vi "Process.vi"(8 "error in (no error)":errorcluster, 10 "Pound in":refnum<class "Pound.lvclass">, 11 "Qbus in":refnum<class "Qbus.lvclass">) -> (0 "error out":errorcluster)   [LabVIEW 2017, in "CmsAnalysis.lvlib"]
doc: "The Analysis process calculates features and spectral bands, or trends, from waveforms the channels in a data group acquire. After these values are calculated, subsequent processes that evaluate their data to trigger alarms, file collections, and so on can operate."
uses:
  <vilib>/addons/InsightCM/Devices/Shared/Cms/CmsAnalysis/CmsAnalysis.lvlib
  <vilib>/addons/Qbus/Qbus.lvclass
  <vilib>/NI/Software Watchdog/Pound/Pound.lvclass
  <vilib>/addons/InsightCM/Devices/Shared/Cms/CmsAnalysis/controls/Config.ctl
  <vilib>/addons/InsightCM/Devices/Shared/Cms/CmsAnalysis/controls/Group.ctl
  <vilib>/addons/InsightCM/Utilities/Analysis/Shared/controls/Channel.ctl
  <vilib>/addons/InsightCM/Utilities/Analysis/Shared/controls/SpeedType.ctl
  <vilib>/addons/InsightCM/Utilities/Analysis/Shared/controls/Feature.ctl
  <vilib>/addons/InsightCM/Utilities/Analysis/Shared/controls/AmplitudeScale.ctl
  <vilib>/NI/Software Watchdog/Watchdog/Watchdog.lvclass
  <vilib>/addons/InsightCM/Devices/Shared/Common/DataFlow/DataFlow.lvlib
  <vilib>/addons/InsightCM/Utilities/Analysis/Shared/AnalysisHelper.lvlib
  <vilib>/addons/InsightCM/Utilities/GlobalConfiguration/GlobalConfiguration.lvlib
  <vilib>/addons/InsightCM/Devices/Shared/Common/DataEventCreator/DataEventCreator.lvlib
  <vilib>/addons/TraceLogger/TraceLogger.lvlib
  <vilib>/addons/InsightCM/Devices/Shared/Cms/CmsDataEventCreator/CmsDataEventCreator.lvlib
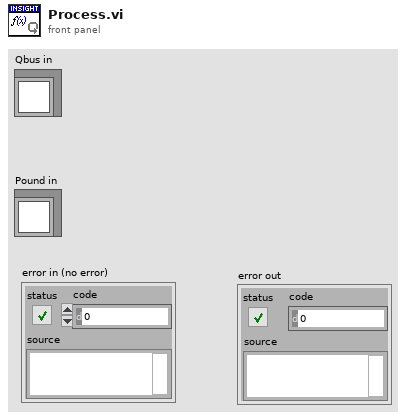
[diagram p1: front panel]
types:
  T1 = typedef "CmsAnalysis.lvlib/Config.ctl" = cluster{"Groups":T2[]}
  T2 = typedef "CmsAnalysis.lvlib/Group.ctl" = cluster{"Name":string, "Channels":T3[]}
  T3 = typedef "AnalysisHelper.lvlib/Channel.ctl" = cluster{"Name":string, "Id":string, "Type":string, "Status Tag":string, "Speed Type":T4, "Speed Reference":string, "Nominal Speed":dbl, "Speed Ratio":dbl, "Pair Channel":string, "Source Channel":string, "Sensitivity":dbl, "Features":T5[], "Acq Timestamp":timestamp}
  T4 = typedef "AnalysisHelper.lvlib/SpeedType.ctl" = enum16{"Fixed Speed", "Tachometer", "From Map"}
  T5 = typedef "AnalysisHelper.lvlib/Feature.ctl" = cluster{"MetricType":string, "TdmsPropName":string, "DisplayName":string, "Unit":string, "Use Volts":bool, "Value":dbl, "Tag Id":string, "Properties":variant, "Amplitude Scale":T6, "valid":bool}
  T6 = typedef "AnalysisHelper.lvlib/AmplitudeScale.ctl" = enum16{"rms", "peak", "pk-pk"}
  T7 = typedef "DataEventCreator.lvlib/RegisterTrendPoints.ctl" = cluster{"DataGroup":string, "Trends":T8[]}
  T8 = typedef "DataEventCreator.lvlib/Registry_Trend.ctl" = cluster{"TrendPointId":string, "DataSetName":string, "HighRate":bool, "Always Send":bool}
  T9 = typedef "DataFlow.lvlib/Data.ctl" = cluster{"DataGroup":string, "Waveforms":T10, "Map":T11, "Type":T12}
  T10 = typedef "wfmSGL_DVR.ctl" = refnum<data-value>
  T11 = typedef "PointValueMap.lvlib/PointMap.ctl" = refnum<data-value>
  T12 = typedef "DataFlow.lvlib/Type.ctl" = enum16{"High Rate", "Low Rate", "Burst Mode"}
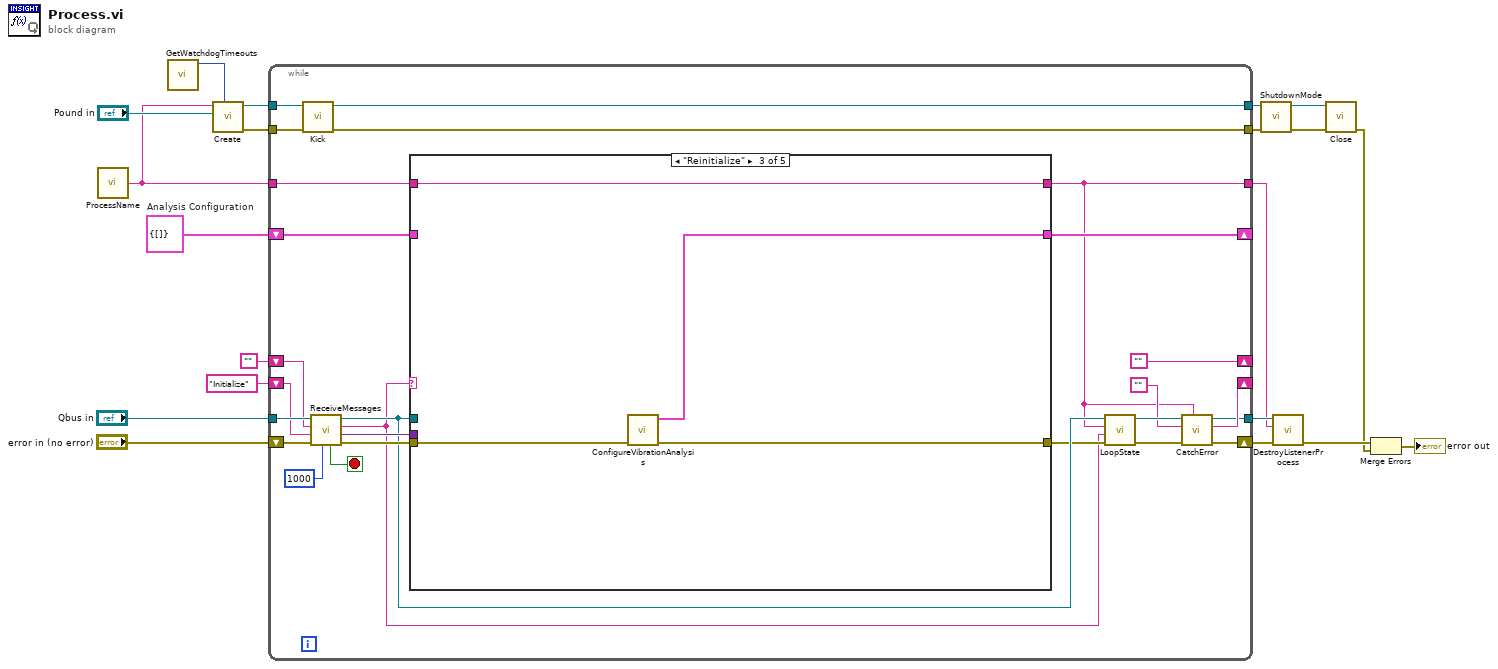
[diagram p0: block diagram]
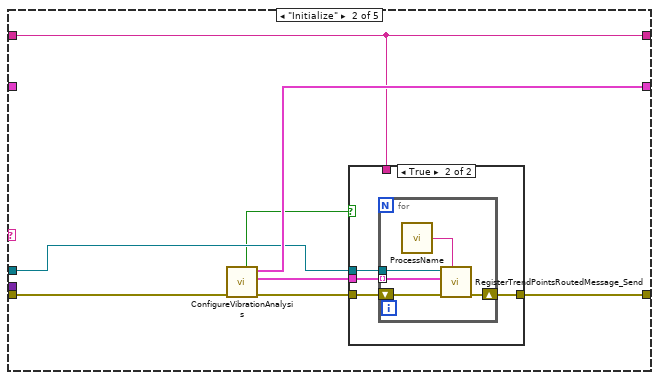
[diagram p3: hidden frame]
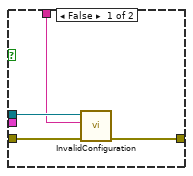
[diagram p4: hidden frame]
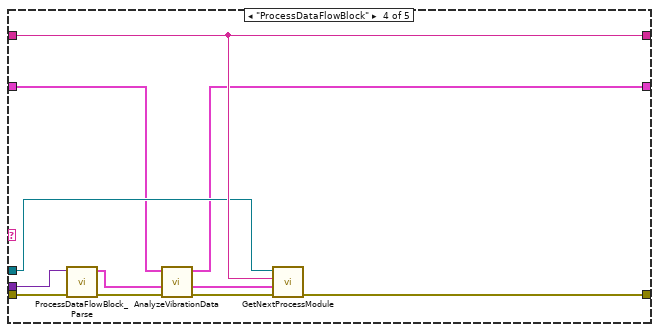
[diagram p5: hidden frame]
diagram:
  w8 = T1 {"Groups"=[]}  # Analysis Configuration
  n1 = call <vilib>:"ProcessName.vi"() -> ("ProcessName"=w13:string)  [unwired: 5 in]
  n2 = call <vilib>:"GetWatchdogTimeouts.vi"() -> ("software timeout"=w1:u32)  [unwired: 10 in, 1 out]
  n3 = call <vilib>:"Create.vi"("Execution Timeout (ms)"=w1, "Pound"="Pound in", "Name"=w13) -> ("error out"=w9:errorcluster, "Watchdog"=w10:refnum<data-value>)  [unwired: 7 in]
  n4 = while {
    shift-right: [""] -> _
    shift-left: "" -> [w40]
    shift-right: [w46] -> _
    shift-left: w8 -> [w45]
    shift-right: [w27] -> _
    shift-left: "Initialize" ("MsgName") -> [w38]
    tunnel: w13 -> [w33]
    tunnel: [w26] -> w16
    tunnel: [w24] -> w15
    tunnel: "Qbus in" -> [w43]
    tunnel: [w37] -> w12
    tunnel: [w36] -> w11
    tunnel: w10 -> [w35]
    tunnel: w9 -> [w34]
    shift-right: [w25] -> w17
    shift-left: "error in (no error)" -> [w39]
    stop <- w22 stop-if-true
    n5 = call <vilib>:"Kick.vi"("error in (no error)"=w34, "Watchdog"=w35) -> ("error out"=w37:errorcluster, "Watchdog"=w36:refnum<data-value>)  [unwired: 8 in]
    n6 = call <vilib>:"ReceiveMessages.vi"("Timeout(100)"=1000, "error in (no error)"=w39, "Priority Action"=w38, "Default Action"=w40, "Qbus in"=w43) -> ("error out"=w41:errorcluster, "MsgValue"=w42:variant, "Action"=w23:string, "Qbus out"=w32:refnum<class "Qbus.lvclass">, "Exit"=w22:bool)  [unwired: 2 in]
    n7 = case shown="\"Reinitialize\"" w23 {
      tunnel: w41 -> [w49 w53 w73 w85 w87]
      tunnel: [w49 w52 w71 w82 w87] -> w31
      tunnel: w42 -> [_ _ _ w84 _]
      tunnel: [w48 w57 w74 w77 w86] -> w46
      tunnel: w45 -> [w48 _ _ w80 w86]
      tunnel: w32 -> [_ w56 _ w81 _]
      tunnel: [w47 w50 w72 w83 w88] -> w24
      tunnel: w33 -> [w47 w50 w72 w83 w88]
      frame Default {
      }
      frame "Initialize" {
        n8 = call <vilib>:"ConfigureVibrationAnalysis.vi"("error in (no error)"=w53) -> ("error out"=w54:errorcluster, "register trends"=w55:T7[], "analysis config"=w57:T1, "valid config"=w51:bool)  [unwired: 7 in]
        n9 = case shown="True" w51 {
          tunnel: w56 -> [w61 w65]
          tunnel: w55 -> [_ w64]
          tunnel: w54 -> [w60 w63]
          tunnel: [w59 w62] -> w52
          tunnel: w50 -> [w58 _]
          frame False {
            n10 = call <vilib>:"InvalidConfiguration.vi"("error in (no error)"=w60, "description"=w58, "Qbus in"=w61) -> ("error out"=w59:errorcluster)  [unwired: 7 in, 1 out]
          }
          frame True {
            n11 = for {
              tunnel: w64 -> [w70] mode=indexing
              shift-right: [w68] -> w62
              shift-left: w63 -> [w69]
              tunnel: w65 -> [w67]
              n12 = call <vilib>:"ProcessName.vi"() -> ("process name"=w66:string)  [unwired: 5 in]
              n13 = call <vilib>:"RegisterTrendPointsRoutedMessage_Send.vi"("data event creator process name"=w66, "error in (no error)"=w69, "register trend"=w70, "Qbus in"=w67) -> ("error out"=w68:errorcluster)  [unwired: 6 in, 1 out]
            }
          }
        }
      }
      frame "Reinitialize" {
        n14 = call <vilib>:"ConfigureVibrationAnalysis.vi"("error in (no error)"=w73) -> ("error out"=w71:errorcluster, "analysis config"=w74:T1)  [unwired: 7 in, 2 out]
      }
      frame "ProcessDataFlowBlock" {
        n15 = call <vilib>:"ProcessDataFlowBlock_Parse.vi"("error in (no error)"=w85, "body"=w84) -> ("error out"=w78:errorcluster, "data"=w79:T9)  [unwired: 8 in]
        n16 = call <vilib>:"AnalyzeVibrationData.vi"("error in (no error)"=w78, "data in"=w79, "Analysis Config"=w80) -> ("error out"=w75:errorcluster, "data out"=w76:T9, "Analysis Config Out"=w77:T1)  [unwired: 6 in]
        n17 = call <vilib>:"GetNextProcessModule.vi"("error in (no error)"=w75, "data"=w76, "source"=w83, "Qbus in"=w81) -> ("error out"=w82:errorcluster)  [unwired: 6 in, 1 out]
      }
      frame "Exit" {
      }
    }
    n18 = call <vilib>:"LoopState.vi"("error in (no error)"=w31, "loop action"=w23, "process name"=w24, "Qbus in"=w32) -> ("error out"=w28:errorcluster, "Qbus out"=w30:refnum<class "Qbus.lvclass">)  [unwired: 6 in]
    n19 = call <vilib>:"CatchError.vi"("source"=w24, "error in (no error)"=w28, "next action in"="", "Qbus in"=w30) -> ("error out"=w25:errorcluster, "next action out"=w27:string, "Qbus out"=w26:refnum<class "Qbus.lvclass">)  [unwired: 5 in]
  }
  n20 = call <vilib>:"ShutdownMode.vi"("error in (no error)"=w12, "Watchdog"=w11) -> ("error out"=w18:errorcluster, "Watchdog"=w19:refnum<data-value>)  [unwired: 8 in]
  n21 = call <vilib>:"DestroyListenerProcess.vi"("error in (no error)"=w17, "process name"=w15, "Qbus in"=w16) -> ("error in (no error)"=w7:errorcluster)  [unwired: 7 in, 1 out]
  n22 = call <vilib>:"Close.vi"("error in (no error)"=w18, "Watchdog"=w19) -> ("error out"=w6:errorcluster)  [unwired: 9 in]
  n23 = Merge Errors(w7, w6) -> (→"error out":errorcluster)
